vi "Handle Drag Starting.vi"(4 "Mods":cluster{"Double Click":bool, "Menu Key":bool}, 5 "Drag Mode":enum32{"copy or move", "copy only", "move only"}(ring), 6 "PlatMods":T3, 7 "Button":u16, 8 "error in (no error)":errorcluster, 9 "Coords":T2, 10 "Data":T4(array[cluster]), 11 "Process Builder View in":refnum<class "Process Builder View.lvclass">) -> (0 "error out":errorcluster, 2 "Drag Starting Filtered Event Data":T1, 3 "Process Builder View out":refnum<class "Process Builder View.lvclass">)   [LabVIEW 2019, in "Process Builder View.lvclass"]
uses:
  <vilib>/gpm_packages/@cs/Car-wash/Source/Process Builder View/Process Builder View.lvclass
  C:/Program Files/National Instruments/LabVIEW 2019/vi.lib/gpm_packages/@cs/Test-executive-builder/Source/Test Executive Builder View/Test Executive Builder View/Test Executive Builder View.lvclass
  <vilib>/Utility/miscctls.llb/LVPoint32TypeDef.ctl
  <vilib>/gpm_packages/@cs/Test-executive-builder/Source/Application Dependencies/Drag Starting Filtered Event Data.ctl
  <vilib>/gpm_packages/@cs/Test-executive-builder/Source/Test Executive Builder View/Test Executive Builder View/Test Executive Builder View.lvclass/Test Executive Builder View.ctl
  <vilib>/gpm_packages/@cs/Test-executive-builder/Source/Test Executive Builder View/Tree Click Interpreter/Tree Click Interpreter.lvclass
  <vilib>/gpm_packages/@cs/Test-executive-builder/Source/Test Executive Builder View/Test Executive Builder View/Test Executive Builder View.lvclass
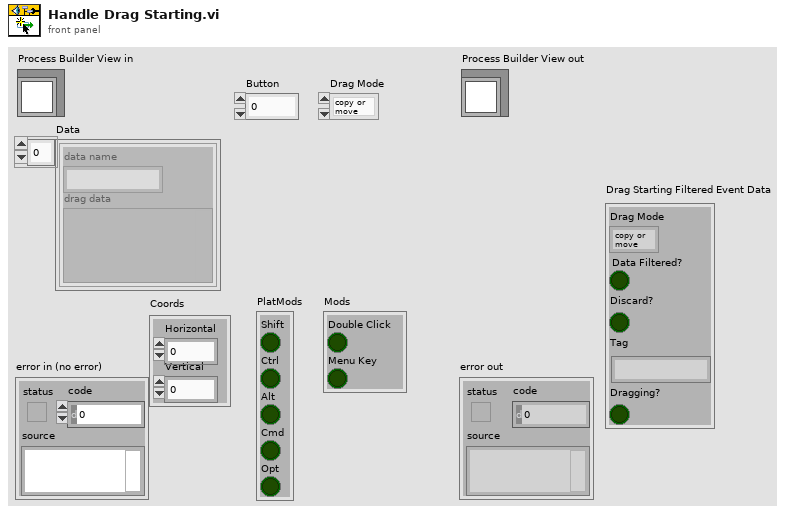
[diagram p1: front panel]
types:
  T1 = typedef "Drag Starting Filtered Event Data.ctl" = cluster{"Drag Mode":enum32{"copy or move", "copy only", "move only"}, "Data Filtered?":bool, "Discard?":bool, "Tag":string, "Dragging?":bool}
  T2 = typedef "LVPoint32TypeDef.ctl" = cluster{"Horizontal":i32, "Vertical":i32}
  T3 = cluster{"Shift":bool, "Ctrl":bool, "Alt":bool, "Cmd":bool, "Opt":bool}
  T4 = cluster{"data name":string, "drag data":variant}[]
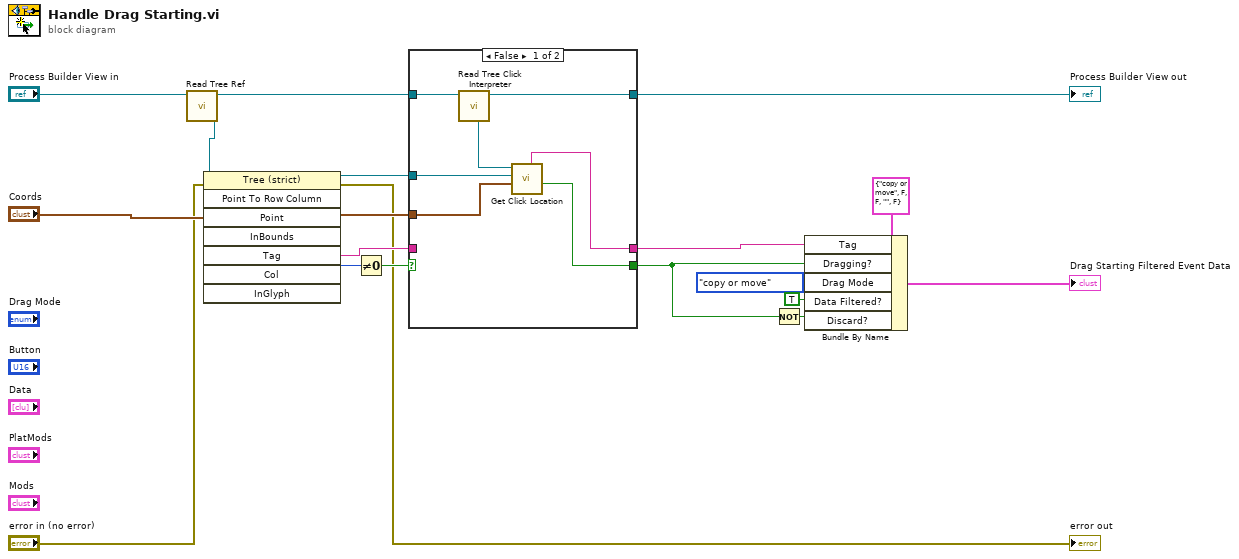
[diagram p0: block diagram]
diagram:
  n1 = call <vilib>:"Read Tree Ref.vi"("Test Executive Builder View in"="Process Builder View in") -> ("Tree Ref"=w17:refnum<vi>, "Test Executive Builder View out"=w10:refnum<class "Process Builder View.lvclass">)  [unwired: 9 in]
  n2 = invoke class="Tree (strict)" method="Point To Row Column"(reference=w17, error in="error in (no error)", "Point"="Coords") -> (reference out=w13:refnum<vi>, error out=→"error out":errorcluster, "Tag"=w14:string, "Col"=w16:i32)  [unwired: 5 in, 4 out]
  n3 = Not Equal To 0?(x=w16) -> (x != 0?=w15:bool)
  n4 = case shown="False" w15 {
    selector: w15 -> [_ w28]
    tunnel: w14 -> [_ w27]
    tunnel: "Coords" -> [w21 _]
    tunnel: w13 -> [w22 _]
    tunnel: [w19 w28] -> w7
    tunnel: [w20 w27] -> w8
    tunnel: [w24 w26] -> w5
    tunnel: w10 -> [w25 w26]
    frame False {
      n5 = call <vilib>:"Read Tree Click Interpreter.vi"("Test Executive Builder View in"=w25) -> ("Test Executive Builder View out"=w24:refnum<class "Process Builder View.lvclass">, "Tree Click Interpreter"=w23:refnum<class "Tree Click Interpreter.lvclass">)  [unwired: 9 in]
      n6 = call-dynamic "Get Click Location.vi"("Coords"=w21, "Tree Refnum"=w22, "Tree Click Interpreter in"=w23) -> ("Valid?"=w19:bool, "Tag"=w20:string)  [unwired: 4 in, 3 out]
    }
    frame True {
    }
  }
  "Process Builder View out" <- w5
  n7 = Not(x=w7) -> (.not. x?=w9:bool)
  n8 = Bundle By Name(cluster=T1 {"Drag Mode"=enum."copy or move", "Data Filtered?"=FALSE, "Discard?"=FALSE, "Tag"="", "Dragging?"=FALSE} ("Drag Starting Filtered Event Data"), "Tag"=w8, "Dragging?"=w7, "Drag Mode"=enum32{"copy or move", "copy only", "move only"}."copy or move", "Data Filtered?"=TRUE, "Discard?"=w9) -> (→"Drag Starting Filtered Event Data":T1)
